vi "script.vi"() -> ()   [LabVIEW 2021]
panel:
  out "appended array":errorcluster[](array[cluster])
  out "Array 6":string[](array[string])
  out "Array 5":string[](array[string])
  out "Array 4":string[](array[string])
  out "Array 3":string[](array[string])
  out "VI Name 4":string
  out "Array 2":string[](array[string])
  out "Array":string[](array[string])
  out "VI Name 3":string
  out "VI Name 2":string
  out "VI Name":string
  out "Application:All VIs In Memory 2":string[](array[string])
  out "Application:All VIs In Memory":string[](array[string])
  out "error out":errorcluster
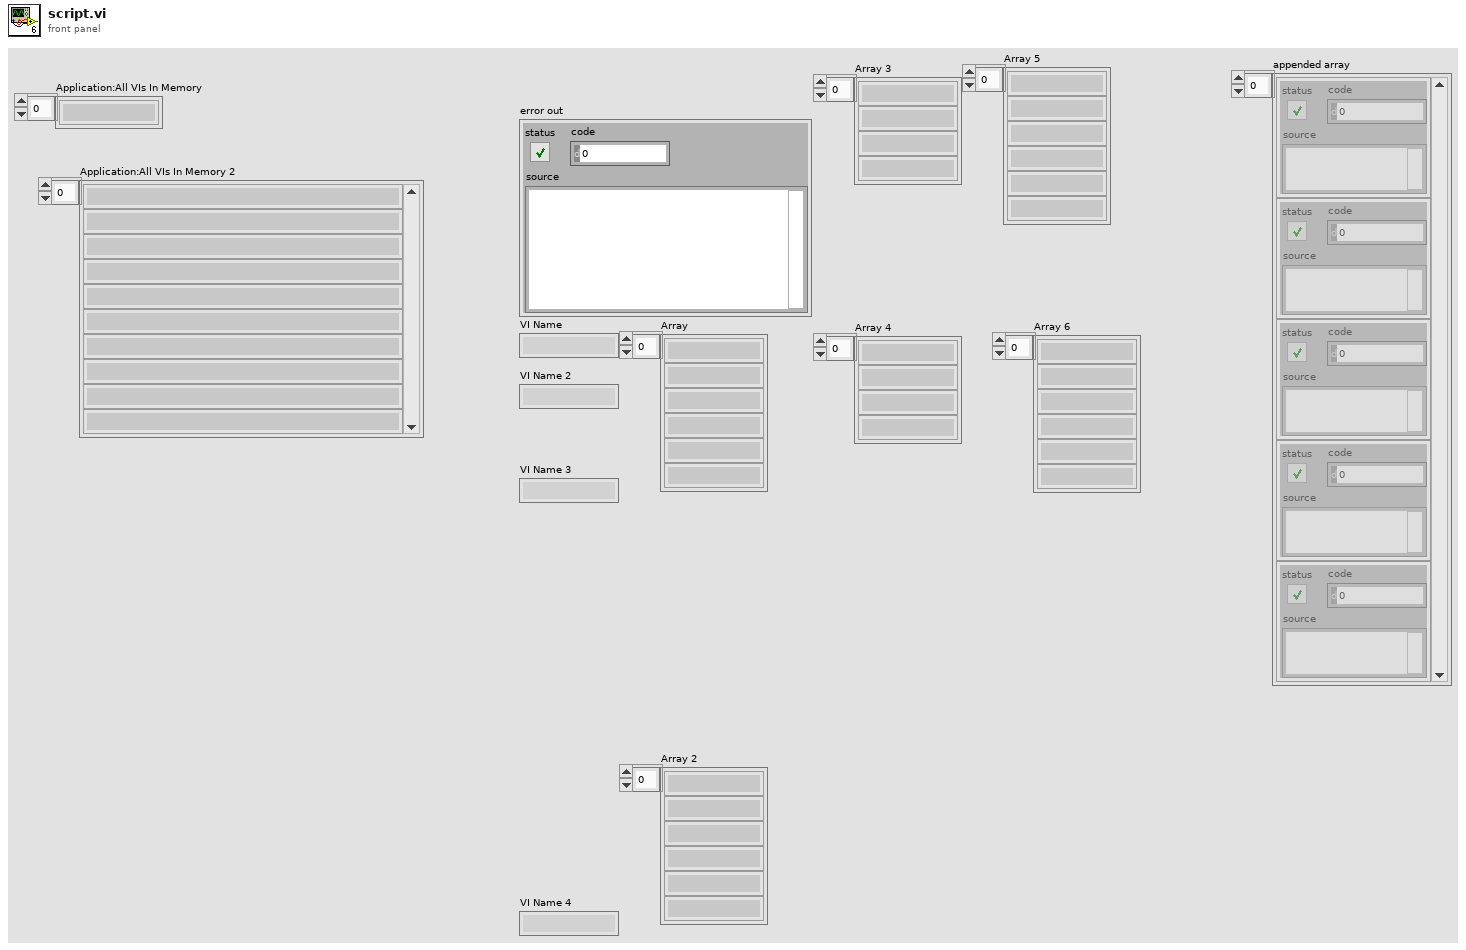
[diagram p1: front panel]
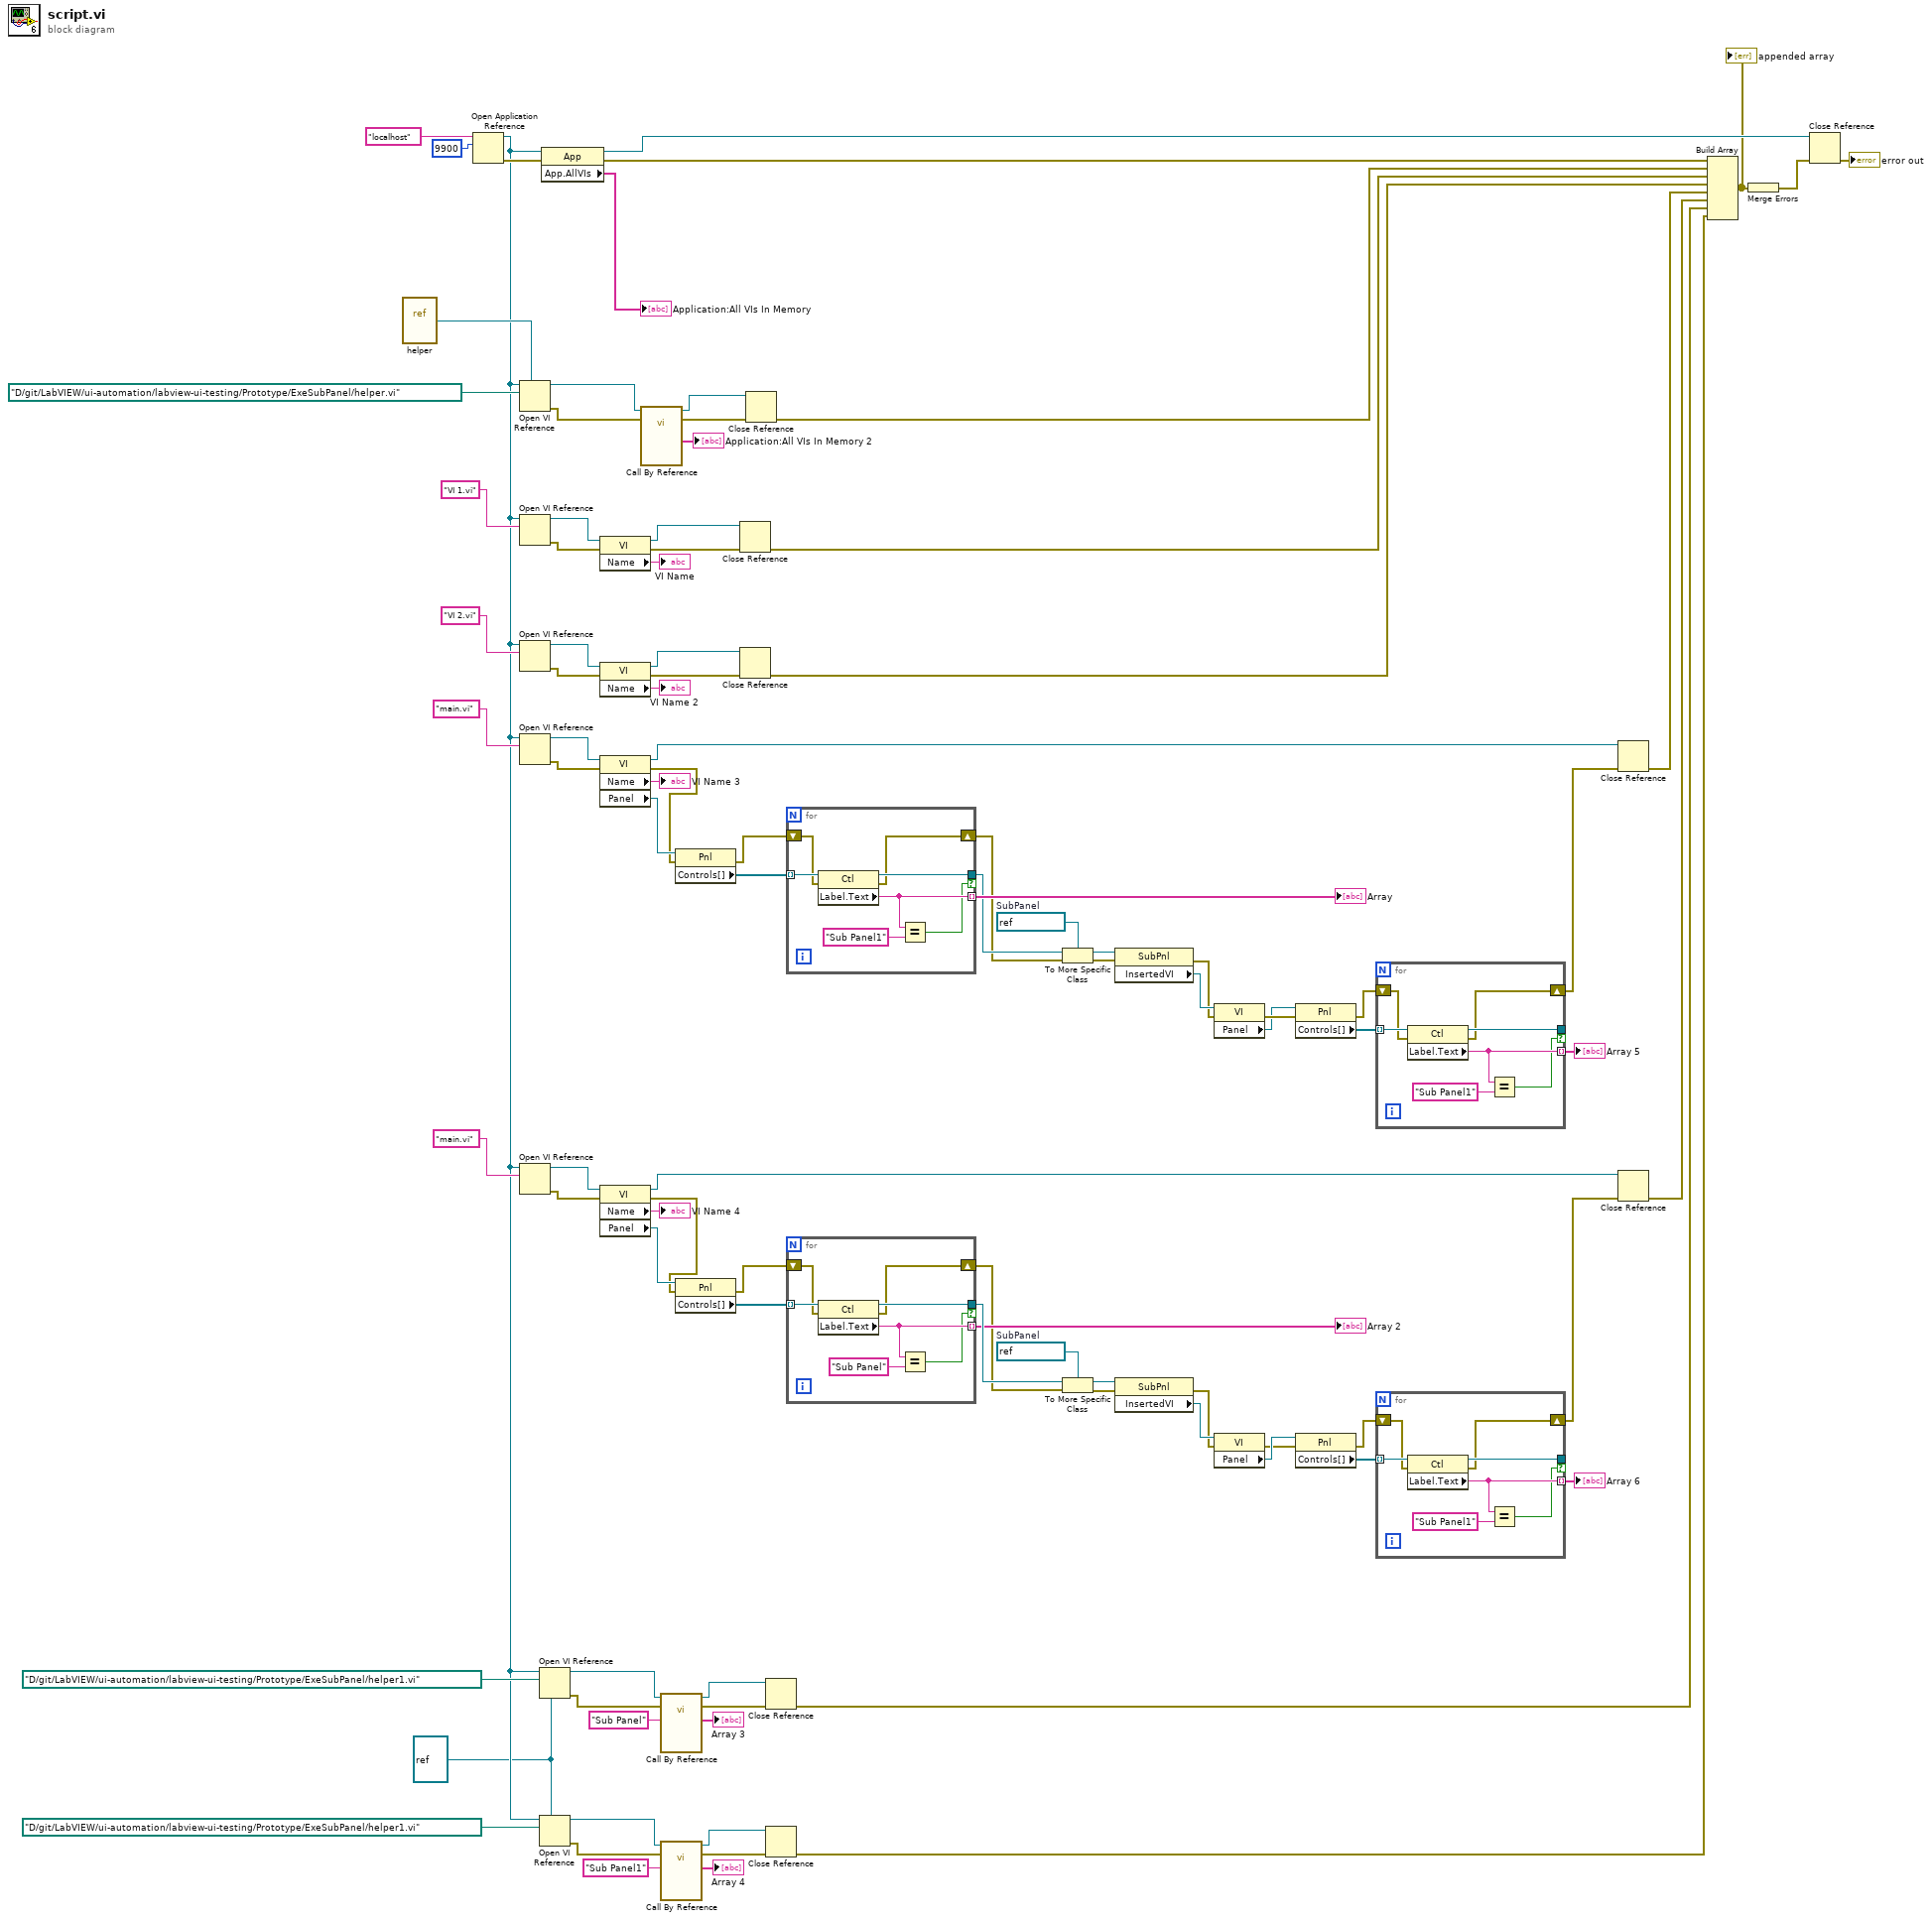
[diagram p0: block diagram]
diagram:
  w2 = refnum<vi> refnum
  w45 = refnum<vi> refnum  # SubPanel
  w56 = refnum<vi> refnum  # SubPanel
  n1 = vi-ref "helper.vi"() -> (w89:refnum<vi>)
  n2 = Open Application Reference(10:u16 9900 ("port number or service name (3363)"), 11:"localhost" ("machine name (\"\":  open local reference)")) -> (0:w95:errorcluster, 3:w17:refnum<vi>)  [unwired: 2 in]
  n3 = Open VI Reference(type specifier VI Refnum (for type only)=w89, application reference (local)=w17, vi path=path "D:/git/LabVIEW/ui-automation/labview-ui-testing/Prototype/ExeSubPanel/helper.vi") -> (vi reference=w88:refnum<vi>, error out=w87:errorcluster)  [unwired: 3 in]
  n4 = Open VI Reference(application reference (local)=w17, vi path="VI 1.vi" ("machine name (\"\":  open local reference)")) -> (vi reference=w79:refnum<vi>, error out=w80:errorcluster)  [unwired: 4 in]
  n5 = Open VI Reference(application reference (local)=w17, vi path="VI 2.vi" ("machine name (\"\":  open local reference)")) -> (vi reference=w71:refnum<vi>, error out=w70:errorcluster)  [unwired: 4 in]
  n6 = Open VI Reference(application reference (local)=w17, vi path="main.vi" ("machine name (\"\":  open local reference)")) -> (vi reference=w65:refnum<vi>, error out=w66:errorcluster)  [unwired: 4 in]
  n7 = Open VI Reference(application reference (local)=w17, vi path="main.vi" ("machine name (\"\":  open local reference)")) -> (vi reference=w37:refnum<vi>, error out=w36:errorcluster)  [unwired: 4 in]
  n8 = Open VI Reference(type specifier VI Refnum (for type only)=w2, application reference (local)=w17, vi path=path "D:/git/LabVIEW/ui-automation/labview-ui-testing/Prototype/ExeSubPanel/helper1.vi") -> (vi reference=w32:refnum<vi>, error out=w31:errorcluster)  [unwired: 3 in]
  n9 = Open VI Reference(type specifier VI Refnum (for type only)=w2, application reference (local)=w17, vi path=path "D:/git/LabVIEW/ui-automation/labview-ui-testing/Prototype/ExeSubPanel/helper1.vi") -> (vi reference=w20:refnum<vi>, error out=w21:errorcluster)  [unwired: 3 in]
  n10 = property class="App"(reference=w17, error in=w95) -> (reference out=w93:refnum<vi>, error out=w94:errorcluster, "App.AllVIs"=→"Application:All VIs In Memory":string[])
  n11 = property class="VI"(reference=w79, error in=w80) -> (reference out=w77:refnum<vi>, error out=w78:errorcluster, "Name"=→"VI Name":string)
  n12 = property class="VI"(reference=w71, error in=w70) -> (reference out=w73:refnum<vi>, error out=w72:errorcluster, "Name"=→"VI Name 2":string)
  n13 = property class="VI"(reference=w65, error in=w66) -> (reference out=w64:refnum<vi>, error out=w8:errorcluster, "Name"=→"VI Name 3":string, "Panel"=w61:refnum<vi>)
  n14 = property class="VI"(reference=w37, error in=w36) -> (reference out=w38:refnum<vi>, error out=w9:errorcluster, "Name"=→"VI Name 4":string, "Panel"=w40:refnum<vi>)
  n15 = call-by-ref "?"(reference=w88, error in=w87) -> (reference out=w85:refnum<vi>, error out=w86:errorcluster, "Application:All VIs In Memory"=→"Application:All VIs In Memory 2":string[])  [unwired: 10 in, 1 out]
  n16 = call-by-ref "?"(reference=w32, error in=w31, "y"="Sub Panel") -> (reference out=w29:refnum<vi>, error out=w30:errorcluster, "Array"=→"Array 3":string[])  [unwired: 9 in, 1 out]
  n17 = call-by-ref "?"(reference=w20, error in=w21, "y"="Sub Panel1") -> (reference out=w23:refnum<vi>, error out=w22:errorcluster, "Array"=→"Array 4":string[])  [unwired: 9 in, 1 out]
  n18 = property class="Pnl"(reference=w61, error in=w8) -> (error out=w7:errorcluster, "Controls[]"=w60:refnum<vi>[])  [unwired: 1 out]
  n19 = property class="Pnl"(reference=w40, error in=w9) -> (error out=w10:errorcluster, "Controls[]"=w41:refnum<vi>[])  [unwired: 1 out]
  n20 = Close Reference(reference=w77, error in (no error)=w78) -> (error out=w75:errorcluster)
  n21 = Close Reference(reference=w73, error in (no error)=w72) -> (error out=w68:errorcluster)
  n22 = Close Reference(reference=w85, error in (no error)=w86) -> (error out=w83:errorcluster)
  n23 = Close Reference(reference=w29, error in (no error)=w30) -> (error out=w26:errorcluster)
  n24 = Close Reference(reference=w23, error in (no error)=w22) -> (error out=w18:errorcluster)
  n25 = for {
    tunnel: w60 -> [w104] mode=indexing
    tunnel: [w103] -> w59 mode=indexing
    shift-right: [w98] -> w6
    shift-left: w7 -> [w99]
    tunnel: [w101] -> w58 if=w100
    n26 = property class="Ctl"(reference=w104, error in=w99) -> (reference out=w101:refnum<vi>, error out=w98:errorcluster, "Label.Text"=w103:string)
    n27 = Equal?(x=w103, y="Sub Panel1") -> (x = y?=w100:bool)
  }
  "Array" <- w59
  n28 = for {
    tunnel: w41 -> [w111] mode=indexing
    tunnel: [w110] -> w42 mode=indexing
    shift-right: [w105] -> w11
    shift-left: w10 -> [w106]
    tunnel: [w108] -> w43 if=w107
    n29 = property class="Ctl"(reference=w111, error in=w106) -> (reference out=w108:refnum<vi>, error out=w105:errorcluster, "Label.Text"=w110:string)
    n30 = Equal?(x=w110, y="Sub Panel") -> (x = y?=w107:bool)
  }
  "Array 2" <- w42
  n31 = To More Specific Class(target class=w56, reference=w58, error in=w6) -> (specific class reference=w57:refnum<vi>, error out=w5:errorcluster)
  n32 = To More Specific Class(target class=w45, reference=w43, error in=w11) -> (specific class reference=w44:refnum<vi>, error out=w12:errorcluster)
  n33 = property class="SubPnl"(reference=w57, error in=w5) -> (error out=w4:errorcluster, "InsertedVI"=w52:refnum<vi>)  [unwired: 1 out]
  n34 = property class="SubPnl"(reference=w44, error in=w12) -> (error out=w13:errorcluster, "InsertedVI"=w49:refnum<vi>)  [unwired: 1 out]
  n35 = property class="VI"(reference=w52, error in=w4) -> (error out=w53:errorcluster, "Panel"=w51:refnum<vi>)  [unwired: 1 out]
  n36 = property class="VI"(reference=w49, error in=w13) -> (error out=w48:errorcluster, "Panel"=w50:refnum<vi>)  [unwired: 1 out]
  n37 = property class="Pnl"(reference=w51, error in=w53) -> (error out=w3:errorcluster, "Controls[]"=w55:refnum<vi>[])  [unwired: 1 out]
  n38 = property class="Pnl"(reference=w50, error in=w48) -> (error out=w14:errorcluster, "Controls[]"=w46:refnum<vi>[])  [unwired: 1 out]
  n39 = for {
    tunnel: w55 -> [w118] mode=indexing
    tunnel: [w117] -> w16 mode=indexing
    shift-right: [w112] -> w54
    shift-left: w3 -> [w113]
    tunnel: [w115] -> _ if=w114
    n40 = property class="Ctl"(reference=w118, error in=w113) -> (reference out=w115:refnum<vi>, error out=w112:errorcluster, "Label.Text"=w117:string)
    n41 = Equal?(x=w117, y="Sub Panel1") -> (x = y?=w114:bool)
  }
  "Array 5" <- w16
  n42 = for {
    tunnel: w46 -> [w125] mode=indexing
    tunnel: [w124] -> w15 mode=indexing
    shift-right: [w119] -> w47
    shift-left: w14 -> [w120]
    tunnel: [w122] -> _ if=w121
    n43 = property class="Ctl"(reference=w125, error in=w120) -> (reference out=w122:refnum<vi>, error out=w119:errorcluster, "Label.Text"=w124:string)
    n44 = Equal?(x=w124, y="Sub Panel1") -> (x = y?=w121:bool)
  }
  "Array 6" <- w15
  n45 = Close Reference(reference=w64, error in (no error)=w54) -> (error out=w62:errorcluster)
  n46 = Close Reference(reference=w38, error in (no error)=w47) -> (error out=w34:errorcluster)
  n47 = Build Array(w94, w83, w75, w68, w62, w34, w26, w18) -> (w84:errorcluster[])
  "appended array" <- w84
  n48 = Merge Errors(w84) -> (w1:errorcluster)
  n49 = Close Reference(reference=w93, error in (no error)=w1) -> (error out=→"error out":errorcluster)
